vi "Fieldbus_Write_message.vi"(9 "Data":i32, 11 "Message":string) -> (3 "Write":T1)   [LabVIEW 2021]
panel:
  out "Message Output":T1
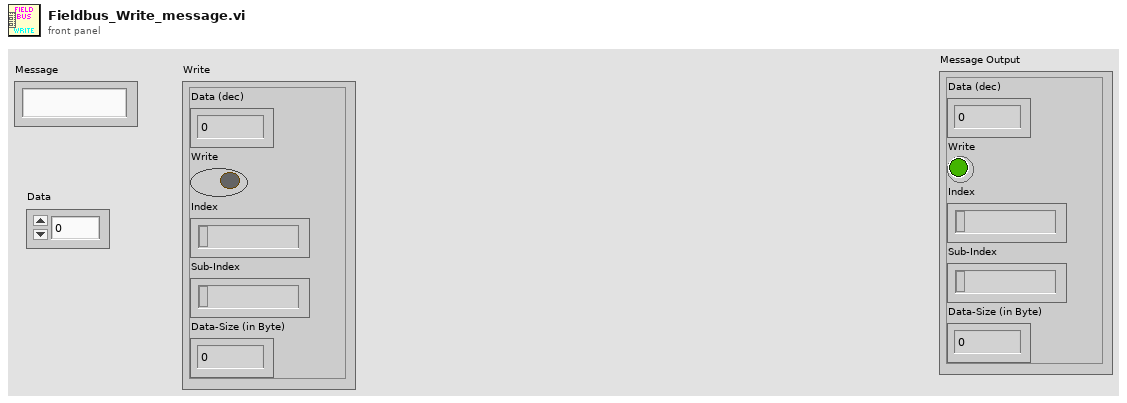
[diagram p1: front panel]
types:
  T1 = cluster{"Data (dec)":i32, "Write":bool, "Index":string, "Sub-Index":string, "Data-Size (in Byte)":u8}
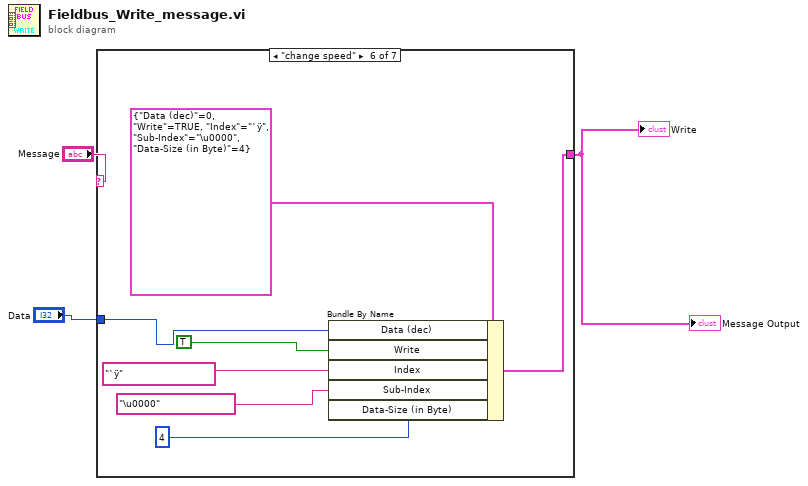
[diagram p0: block diagram]
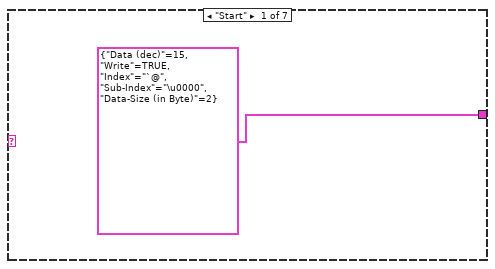
[diagram p2: hidden frame]
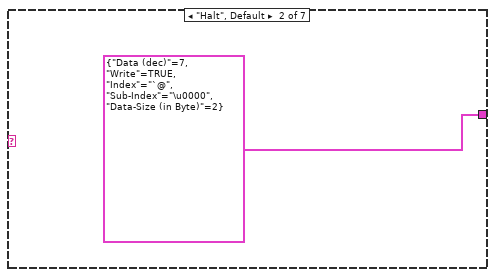
[diagram p3: hidden frame]
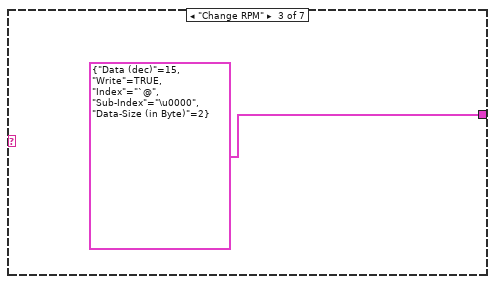
[diagram p4: hidden frame]
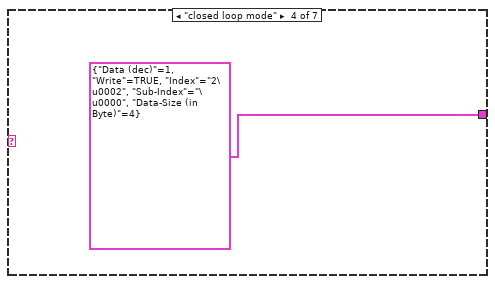
[diagram p5: hidden frame]
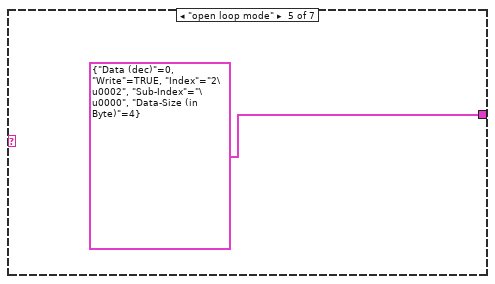
[diagram p6: hidden frame]
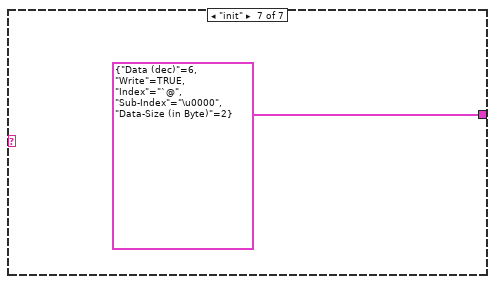
[diagram p7: hidden frame]
diagram:
  n1 = case shown="\"change speed\"" "Message" {
    tunnel: [T1 {"Data (dec)"=15, "Write"=TRUE, "Index"="`@", "Sub-Index"="\u0000", "Data-Size (in Byte)"=2} ("Write") T1 {"Data (dec)"=7, "Write"=TRUE, "Index"="`@", "Sub-Index"="\u0000", "Data-Size (in Byte)"=2} ("Write") T1 {"Data (dec)"=15, "Write"=TRUE, "Index"="`@", "Sub-Index"="\u0000", "Data-Size (in Byte)"=2} ("Write") T1 {"Data (dec)"=1, "Write"=TRUE, "Index"="2\u0002", "Sub-Index"="\u0000", "Data-Size (in Byte)"=4} ("Write") T1 {"Data (dec)"=0, "Write"=TRUE, "Index"="2\u0002", "Sub-Index"="\u0000", "Data-Size (in Byte)"=4} ("Write") w14 T1 {"Data (dec)"=6, "Write"=TRUE, "Index"="`@", "Sub-Index"="\u0000", "Data-Size (in Byte)"=2} ("Write")] -> w3
    tunnel: "Data" -> [_ _ _ _ _ w13 _]
    frame "Start" {
    }
    frame "Halt", Default {
    }
    frame "Change RPM" {
    }
    frame "closed loop mode" {
    }
    frame "open loop mode" {
    }
    frame "change speed" {
      n2 = Bundle By Name(cluster=T1 {"Data (dec)"=0, "Write"=TRUE, "Index"="`ÿ", "Sub-Index"="\u0000", "Data-Size (in Byte)"=4} ("Write"), "Data (dec)"=w13, "Write"=TRUE, "Index"="`ÿ", "Sub-Index"="\u0000", "Data-Size (in Byte)"=u8 4) -> (w14:T1)
    }
    frame "init" {
    }
  }
  "Write" <- w3
  "Message Output" <- w3
